vi "software limit.vi"(1 "variables":T1, 2 "Encoder":T2) -> (0 "limited":bool)   [LabVIEW 2012]
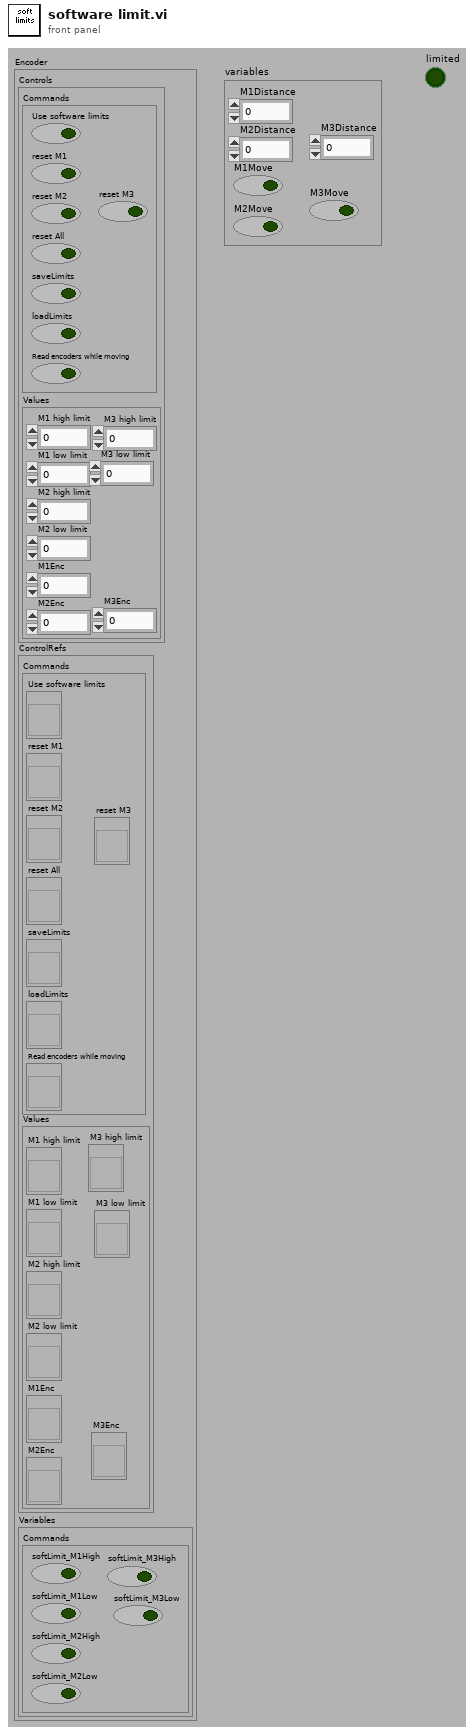
[diagram p1: front panel]
types:
  T1 = cluster{"M1Distance":dbl, "M2Distance":dbl, "M1Move":bool, "M2Move":bool, "M3Distance":dbl, "M3Move":bool}
  T2 = cluster{"Controls":cluster{"Commands":cluster{"Use software limits":bool, "reset M1":bool, "reset M2":bool, "reset All":bool, "saveLimits":bool, "loadLimits":bool, "Read encoders while moving":bool, "reset M3":bool}, "Values":cluster{"M1 high limit":dbl, "M1 low limit":dbl, "M2 high limit":dbl, "M2 low limit":dbl, "M1Enc":dbl, "M2Enc":dbl, "M3 high limit":dbl, "M3 low limit":dbl, "M3Enc":dbl}}, "ControlRefs":cluster{"Commands":cluster{"Use software limits":refnum<vi>, "reset M1":refnum<vi>, "reset M2":refnum<vi>, "reset All":refnum<vi>, "saveLimits":refnum<vi>, "loadLimits":refnum<vi>, "Read encoders while moving":refnum<vi>, "reset M3":refnum<vi>}, "Values":cluster{"M1 high limit":refnum<vi>, "M1 low limit":refnum<vi>, "M2 high limit":refnum<vi>, "M2 low limit":refnum<vi>, "M1Enc":refnum<vi>, "M2Enc":refnum<vi>, "M3 low limit":refnum<vi>, "M3 high limit":refnum<vi>, "M3Enc":refnum<vi>}}, "Variables":cluster{"Commands":cluster{"softLimit_M1High":bool, "softLimit_M1Low":bool, "softLimit_M2High":bool, "softLimit_M2Low":bool, "softLimit_M3High":bool, "softLimit_M3Low":bool}}}
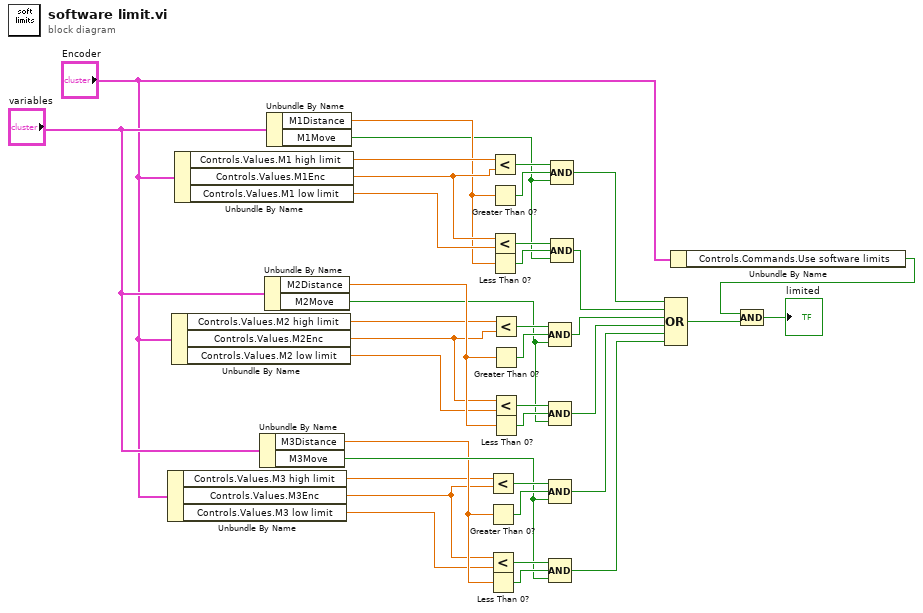
[diagram p0: block diagram]
diagram:
  n1 = Unbundle By Name("Encoder") -> ("Controls.Values.M3 high limit"=w13:dbl, "Controls.Values.M3Enc"=w12:dbl, "Controls.Values.M3 low limit"=w11:dbl)
  n2 = Unbundle By Name("Encoder") -> ("Controls.Values.M2 high limit"=w18:dbl, "Controls.Values.M2Enc"=w17:dbl, "Controls.Values.M2 low limit"=w16:dbl)
  n3 = Unbundle By Name("Encoder") -> ("Controls.Values.M1 high limit"=w25:dbl, "Controls.Values.M1Enc"=w24:dbl, "Controls.Values.M1 low limit"=w23:dbl)
  n4 = Unbundle By Name("variables") -> ("M3Distance"=w14:dbl, "M3Move"=w15:bool)
  n5 = Unbundle By Name("variables") -> ("M2Distance"=w20:dbl, "M2Move"=w19:bool)
  n6 = Unbundle By Name("variables") -> ("M1Distance"=w22:dbl, "M1Move"=w21:bool)
  n7 = Less?(x=w13, y=w12) -> (x < y?=w29:bool)
  n8 = Greater Than 0?(x=w14) -> (x > 0?=w28:bool)
  n9 = Less?(x=w12, y=w11) -> (x < y?=w27:bool)
  n10 = Less Than 0?(x=w14) -> (x < 0?=w26:bool)
  n11 = Less?(x=w25, y=w24) -> (x < y?=w37:bool)
  n12 = Greater Than 0?(x=w22) -> (x > 0?=w36:bool)
  n13 = Less?(x=w24, y=w23) -> (x < y?=w35:bool)
  n14 = Less Than 0?(x=w22) -> (x < 0?=w34:bool)
  n15 = Less?(x=w18, y=w17) -> (x < y?=w33:bool)
  n16 = Greater Than 0?(x=w20) -> (x > 0?=w32:bool)
  n17 = Less?(x=w17, y=w16) -> (x < y?=w31:bool)
  n18 = Less Than 0?(x=w20) -> (x < 0?=w30:bool)
  n19 = Compound Arithmetic op=AND(w33, w32, w19) -> (w8:bool)
  n20 = Compound Arithmetic op=AND(w31, w30, w19) -> (w7:bool)
  n21 = Compound Arithmetic op=AND(w29, w28, w15) -> (w6:bool)
  n22 = Compound Arithmetic op=AND(w27, w26, w15) -> (w5:bool)
  n23 = Compound Arithmetic op=AND(w37, w36, w21) -> (w10:bool)
  n24 = Compound Arithmetic op=AND(w35, w34, w21) -> (w9:bool)
  n25 = Compound Arithmetic op=OR(w10, w9, w8, w7, w6, w5) -> (w4:bool)
  n26 = Unbundle By Name("Encoder") -> ("Controls.Commands.Use software limits"=w3:bool)
  n27 = Compound Arithmetic op=AND(w3, w4) -> (→"limited":bool)
